vi "tc_init.vi"(0 "TC Label":string, 5 "Temperature":dbl format="%#_13g", 7 "Graph ON/OFF":u32(colorbox)=4250624, 9 "Plot Color":u32(colorbox)=16860, 11 "Alarm String":string, 12 "index (row)":i32, 13 "AlarmColor":u32(colorbox)) -> (4 "output array":T1(array[cluster]), 15 "initialized array":bool[](array[boolean]))   [LabVIEW 2017]
panel:
  in  "Boolean":bool
  in  "stop":bool
  in  "index (col)":i32
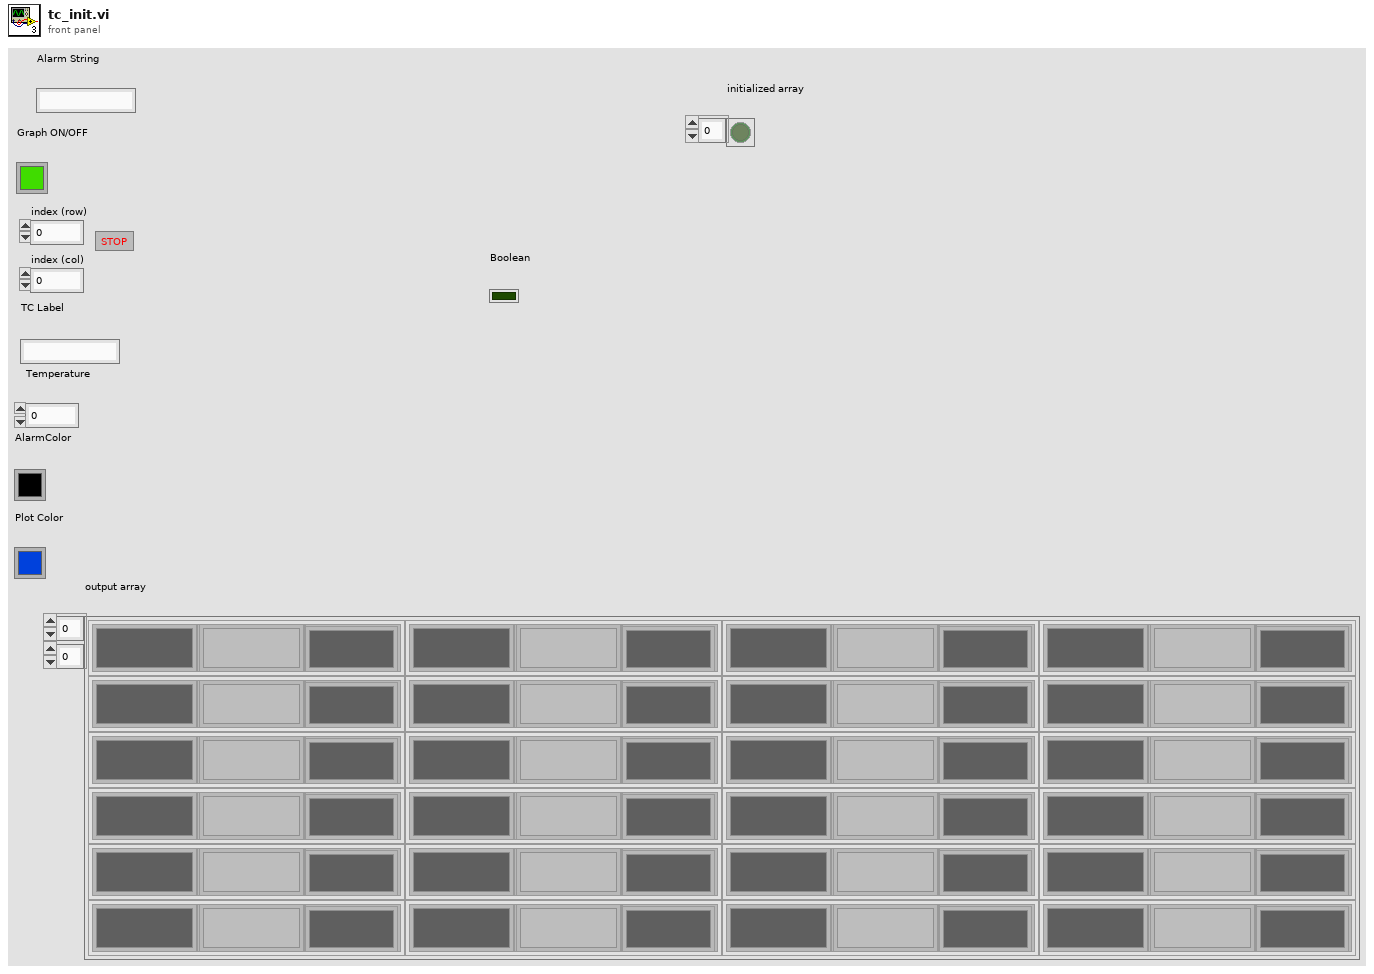
[diagram p1: front panel]
types:
  T1 = cluster{"TC Label":string, "Alarm Status":string, "Alarm Color":u32, "Temperature":string, "PlotColor":u32, "Graph On/Off":u32}[][]
  T2 = cluster{"TC Label":string, "Alarm Status":string, "Alarm Color":u32, "Temperature":string, "PlotColor":u32, "Graph On/Off":u32}
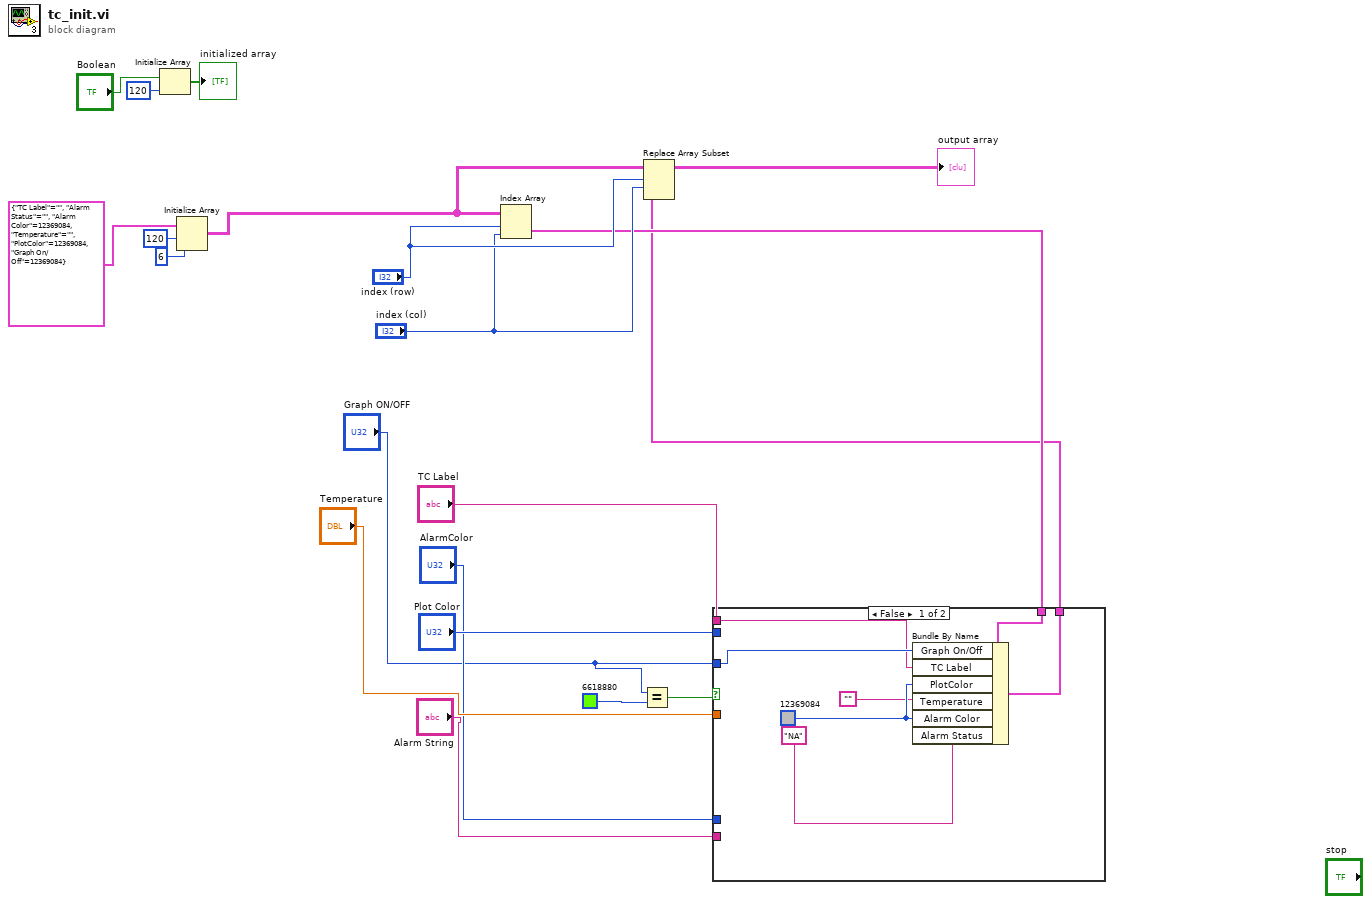
[diagram p0: block diagram]
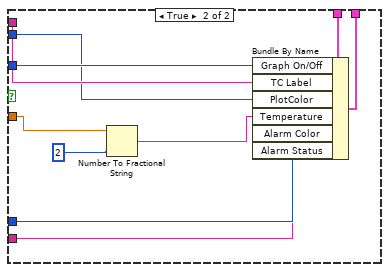
[diagram p2: hidden frame]
diagram:
  n1 = Initialize Array("Boolean", 120 ("dimension size")) -> (→"initialized array":bool[])
  n2 = Initialize Array(T2 {"TC Label"="", "Alarm Status"="", "Alarm Color"=12369084, "Temperature"="", "PlotColor"=12369084, "Graph On/Off"=12369084}, 120 ("dimension size"), 6 ("dimension size")) -> (w18:T1)
  n3 = Index Array(array=w18, index (row)="index (row)", index (col)="index (col)") -> (element=w15:T2)
  n4 = Equal?(x="Graph ON/OFF", y=u32 6618880) -> (x = y?=w6:bool)
  n5 = case shown="False" w6 {
    tunnel: w15 -> [w27 w37]
    tunnel: "Graph ON/OFF" -> [w25 w36]
    tunnel: "TC Label" -> [w22 w35]
    tunnel: "Plot Color" -> [_ w34]
    tunnel: "Temperature" -> [_ w30]
    tunnel: "AlarmColor" -> [_ w33]
    tunnel: "Alarm String" -> [_ w32]
    tunnel: [w26 w31] -> w9
    frame False {
      w23 = u32 12369084 ("Alarm Color")
      n6 = Bundle By Name(cluster=w27, "Graph On/Off"=w25, "TC Label"=w22, "PlotColor"=w23, "Temperature"="", "Alarm Color"=w23, "Alarm Status"="NA") -> (w26:T2)
    }
    frame True {
      n7 = Number To Fractional String(number=w30, precision (6)=i16 2 ("width (-)")) -> (F-format string=w29:string)  [unwired: 2 in]
      n8 = Bundle By Name(cluster=w37, "Graph On/Off"=w36, "TC Label"=w35, "PlotColor"=w34, "Temperature"=w29, "Alarm Color"=w33, "Alarm Status"=w32) -> (w31:T2)
    }
  }
  n9 = Replace Array Subset(array=w18, new element=w9, index (row)="index (row)", index (col)="index (col)") -> (→"output array":T1)
